vi "sub_degminsec.vi"(11 "경위도 (lon, lat)":dbl) -> (2 "도분초":string, 3 "도 (degree)":dbl)   [LabVIEW 2020]
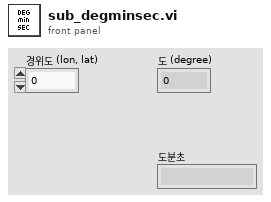
[diagram p1: front panel]
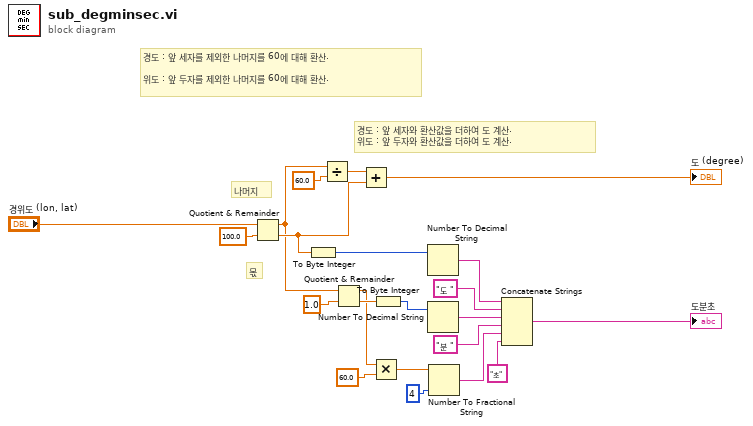
[diagram p0: block diagram]
diagram:
  # "경도 : 앞 세자와 환산값을 더하여 도 계산.\n위도 : 앞 두자와 환산값을 더하여 도 계산."
  # "경도 : 앞 세자를 제외한 나머지를 60에 대해 환산.\n\n위도 : 앞 두자를 제외한 나머지를 60에 대해 환산."
  # "몫"
  # "나머지"
  n1 = Quotient & Remainder(x="경위도 (lon, lat)", y=100.0) -> (x-y*floor(x/y)=w13:dbl, floor(x/y)=w17:dbl)
  n2 = To Byte Integer(number=w17) -> (8bit integer=w16:i8)
  n3 = Divide(x=w13, y=60.0) -> (x/y=w18:dbl)
  n4 = Quotient & Remainder(x=w13, y=1.0) -> (x-y*floor(x/y)=w7:dbl, floor(x/y)=w11:dbl)
  n5 = Add(x=w18, y=w17) -> (x+y=→"도 (degree)":dbl)
  n6 = Multiply(x=w7, y=60.0) -> (x*y=w4:dbl)
  n7 = To Byte Integer(number=w11) -> (8bit integer=w10:i8)
  n8 = Number To Decimal String(number=w16) -> (decimal integer string=w15:string)  [unwired: 1 in]
  n9 = Number To Decimal String(number=w10) -> (decimal integer string=w9:string)  [unwired: 1 in]
  n10 = Number To Fractional String(number=w4, precision (6)=i16 4 ("정밀도(6)")) -> (F-format string=w3:string)  [unwired: 2 in]
  n11 = Concatenate Strings(w15, "도 " ("문자열"), w9, "분 " ("문자열"), w3, "초" ("문자열")) -> (→"도분초":string)
